vi "Test gRPC cRIO XNET Read DBC Signals.vi"(11 "Test Case In":refnum<class "Test Communicator.lvclass">) -> (0 "error out":errorcluster, 3 "Test Case Out":refnum<class "Test Communicator.lvclass">)   [LabVIEW 2024, in "Test Communicator.lvclass"]
uses:
  Test Communicator.lvclass
  Test Communicator.lvclass/Test Communicator.ctl
  Source/Configure Strategies/gRPC XNET Read Raw CAN Frame Strategy/gRPC XNET Read Raw CAN Frame Strategy.lvclass
  <vilib>/Astemes/LUnit/Test Case.lvclass
  Source/DBC Communication/DBC Communication.lvclass
  Source/Communicator/Communicator.lvclass
panel:
  out "Time Stamp":timestamp format="%<%x %.3X>T"
  out "Temp":dbl
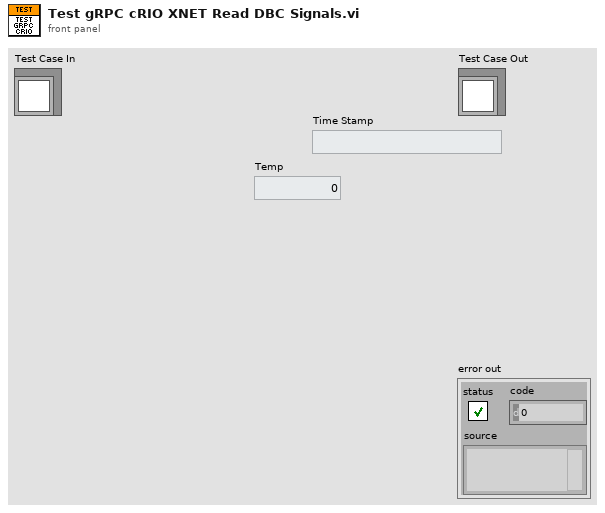
[diagram p1: front panel]
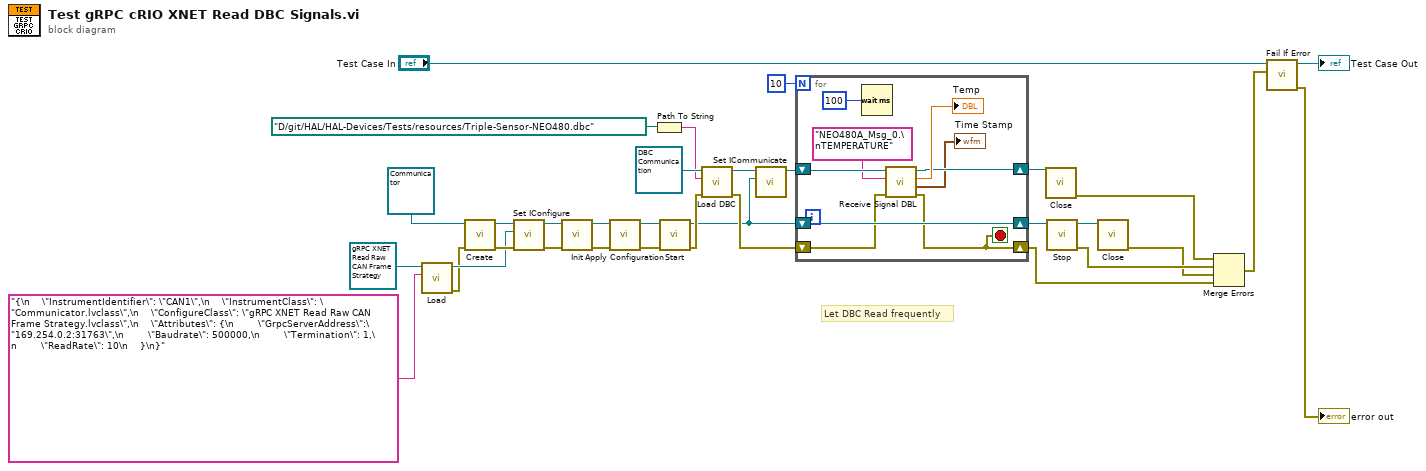
[diagram p0: block diagram]
diagram:
  # "Let DBC Read frequently"
  n1 = call-dynamic "Load.vi"("Source"="{\n    \"InstrumentIdentifier\": \"CAN1\",\n    \"InstrumentClass\": \"Communicator.lvclass\",\n    \"ConfigureClass\": \"gRPC XNET Read Raw CAN Frame Strategy.lvclass\",\n    \"Attributes\": {\n        \"GrpcServerAddress\":\"169.254.0.2:31763\",\n        \"Baudrate\": 500000,\n        \"Termination\": 1,\n        \"ReadRate\": 10\n    }\n}", "gRPC XNET Read Raw CAN Frame Strategy in"=refnum<class "gRPC XNET Read Raw CAN Frame Strategy.lvclass"> refnum ("IConfigure")) -> ("error out"=w15:errorcluster, "gRPC XNET Read Raw CAN Frame Strategy out"=w29:refnum<class "gRPC XNET Read Raw CAN Frame Strategy.lvclass">)  [unwired: 8 in]
  n2 = call-dynamic "Create.vi"("Error In"=w15, "reference in"=refnum<class "Communicator.lvclass"> refnum ("Communicator in")) -> ("Error Out"=w30:errorcluster, "reference out"=w21:refnum<class "Communicator.lvclass">)  [unwired: 8 in]
  n3 = call-dynamic "Set IConfigure.vi"("Error In"=w30, "IConfigure"=w29, "Communicator in"=w21) -> ("Error Out"=w27:errorcluster, "Communicator out"=w26:refnum<class "Communicator.lvclass">)  [unwired: 7 in]
  n4 = call-dynamic "Init.vi"("Error In"=w27, "Communicator in"=w26) -> ("Error Out"=w25:errorcluster, "Communicator out"=w24:refnum<class "Communicator.lvclass">)  [unwired: 8 in]
  n5 = call-dynamic "Apply Configuration.vi"("Error In"=w25, "Communicator in"=w24) -> ("Error Out"=w19:errorcluster, "Communicator out"=w10:refnum<class "Communicator.lvclass">)  [unwired: 8 in]
  n6 = Path To String(path=path "D:/git/HAL/HAL-Devices/Tests/resources/Triple-Sensor-NEO480.dbc") -> (string=w11:string)
  n7 = call-dynamic "Start.vi"("Error In"=w19, "Communicator in"=w10) -> ("Error Out"=w8:errorcluster, "Communicator out"=w4:refnum<class "Communicator.lvclass">)  [unwired: 8 in]
  n8 = call "Load DBC.vi"("error in"=w8, "DBC File"=w11, "DBCCommunication in"=refnum<class "DBC Communication.lvclass"> refnum ("DBC Communication.lvclass")) -> ("error out"=w7:errorcluster, "DBCCommunication out"=w13:refnum<class "DBC Communication.lvclass">)  [unwired: 7 in]
  n9 = call "Set ICommunicate.vi"("ICommunicate"=w4, "DBCCommunication in"=w13) -> ("DBCCommunication out"=w9:refnum<class "DBC Communication.lvclass">)  [unwired: 9 in]
  n10 = for {
    N: 10 -> [_]
    shift-right: [w42] -> w22
    shift-left: w4 -> [w42]
    shift-right: [w34] -> w3
    shift-left: w7 -> [w37]
    shift-right: [w36] -> w6
    shift-left: w9 -> [w40]
    stop <- w34 stop-if-true
    n11 = Wait (ms)(milliseconds to wait=u32 100) -> ()  [unwired: 1 out]
    n12 = call "Receive Signal DBL.vi"("error in"=w37, "Signal Name"="NEO480A_Msg_0.\nTEMPERATURE", "DBC Communication in"=w40) -> ("error out"=w34:errorcluster, "Time Stamp"=→"Time Stamp":timestamp, "Value"=→"Temp":dbl, "DBC Communication out"=w36:refnum<class "DBC Communication.lvclass">)  [unwired: 5 in]
  }
  n13 = call-dynamic "Close.vi"("DBC Communication in"=w6) -> ("error out"=w5:errorcluster)  [unwired: 9 in, 1 out]
  n14 = call-dynamic "Stop.vi"("Communicator in"=w22) -> ("Error Out"=w17:errorcluster, "Communicator out"=w20:refnum<class "Communicator.lvclass">)  [unwired: 9 in]
  n15 = call-dynamic "Close.vi"("Communicator in"=w20) -> ("Error Out"=w1:errorcluster)  [unwired: 9 in, 1 out]
  n16 = Merge Errors(w5, w17, w1, w3) -> (w18:errorcluster)
  n17 = call <vilib>:"Fail If Error.vi"("Assert error"=w18, "LUnit Test Case In"="Test Case In") -> ("error out"=→"error out":errorcluster, "LUnit Test Case Out"=→"Test Case Out":refnum<class "Test Communicator.lvclass">)  [unwired: 8 in]
